vi "GetAnalog.vi"(0 "Connexion réseau UDP en entrée":refnum<k16>, 1 "Pin":u8, 2 "entrée d'erreur (pas d'erreur)":errorcluster, 3 "Adresse IP":u32, 5 "Port Distant":u16) -> (6 "Connexion réseau UDP en sortie":refnum<k16>, 7 "sortie d'erreur":errorcluster, 8 "Return Value":u16)   [LabVIEW 2021]
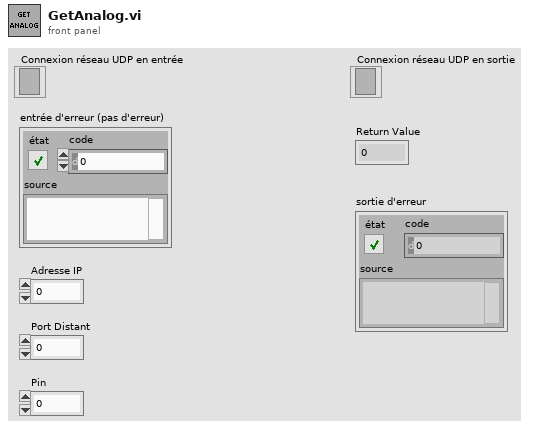
[diagram p1: front panel]
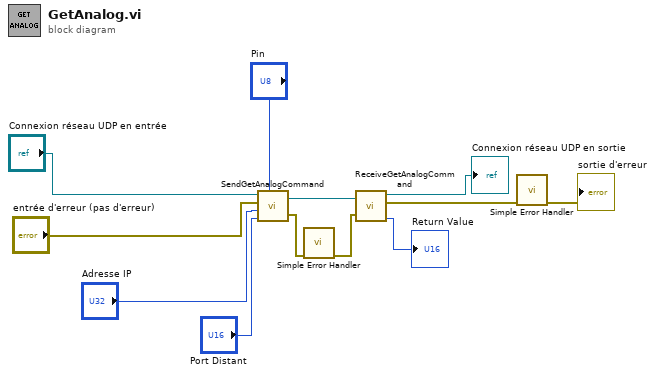
[diagram p0: block diagram]
diagram:
  n1 = call "SendGetAnalogCommand.vi"("Pin"="Pin", "Port Destination"="Port Distant", "Adresse IP Destination"="Adresse IP", "entrée d'erreur"="entrée d'erreur (pas d'erreur)", "Connexion réseau UDP en entrée"="Connexion réseau UDP en entrée") -> ("sortie d'erreur 2"=w1:errorcluster, "Connexion réseau UDP en sortie"=w2:refnum<k16>)  [unwired: 1 in]
  n2 = call <vilib>:"Simple Error Handler.vi"("error in (no error)"=w1) -> ("error out"=w3:errorcluster)  [unwired: 4 in, 4 out]
  n3 = call "ReceiveGetAnalogCommand.vi"("Connexion réseau UDP en entrée"=w2, "entrée d'erreur (pas d'erreur)"=w3) -> ("Connexion réseau UDP en sortie"=→"Connexion réseau UDP en sortie":refnum<k16>, "sortie d'erreur"=w5:errorcluster, "Value"=→"Return Value":u16)  [unwired: 1 out]
  n4 = call <vilib>:"Simple Error Handler.vi"("error in (no error)"=w5) -> ("error out"=→"sortie d'erreur":errorcluster)  [unwired: 4 in, 4 out]
